vi "Stop Histogram Actor.vi"(8 "error in (no error)":errorcluster, 11 "Histogram in":refnum<class "Histogram.lvclass">) -> (0 "error out":errorcluster, 3 "Histogram out":refnum<class "Histogram.lvclass">)   [LabVIEW 2016, in "Tests.lvlib" / "Histogram.lvclass"]
uses:
  Histogram.lvclass
  Histogram.lvclass/Histogram.ctl
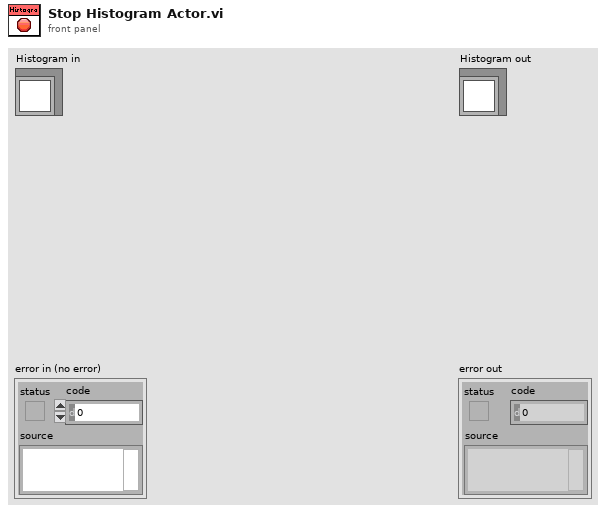
[diagram p1: front panel]
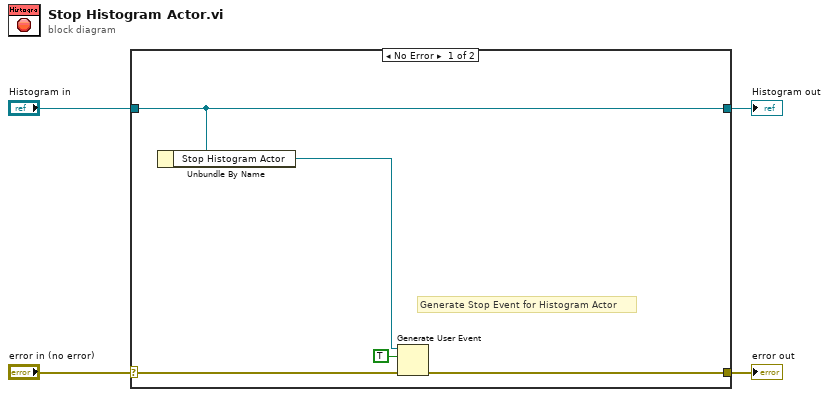
[diagram p0: block diagram]
diagram:
  n1 = case shown="No Error" "error in (no error)" {
    selector: "error in (no error)" -> [w8 w11]
    tunnel: [w7 w11] -> w3
    tunnel: [w9 w10] -> w1
    tunnel: "Histogram in" -> [w9 w10]
    frame No Error {
      # "Generate Stop Event for Histogram Actor"
      n2 = Unbundle By Name(w9) -> ("Stop Histogram Actor"=w6:refnum<user-event>)
      n3 = Generate User Event(user event=w6, event data cluster=TRUE ("event data"), error in=w8) -> (error out=w7:errorcluster)  [unwired: 1 in, 1 out]
    }
    frame Error {
    }
  }
  "error out" <- w3
  "Histogram out" <- w1
